vi "Aux DMA FIFO test.vi"() -> ()   [LabVIEW 2019]
uses:
  <vilib>/rvi/Emulation/niFpgaGetClockAttributes.vi
  <vilib>/rvi/Emulation/niFpgaSctlEmulationGetInTimedLoop.vi
  <vilib>/rvi/Emulation/niFpgaEmulationReportErrorSimple.vi
  <vilib>/rvi/eio/common/nirviEmuTemplateMethod_errors.vi
  <vilib>/rvi/Emulation/niFpgaCriticalErrorInLSC.vi
  <vilib>/rvi/interface/RandomDataEmulation/niFpgaRandomDataHandleErrors.vi
  <vilib>/eio/EIONode/EIONode.xnode
  <vilib>/rvi/DataTransferAndStorage/Container/XNode/niFpgaContainer.xnode
  <vilib>/rvi/interface/RandomDataEmulation/nirviRandomDataFpgaReadWriteTemplate.vi
panel:
  in  "xt end aux":u32
  in  "stop":bool
  out "elapsed":u32
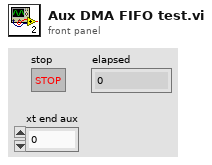
[diagram p1: front panel]
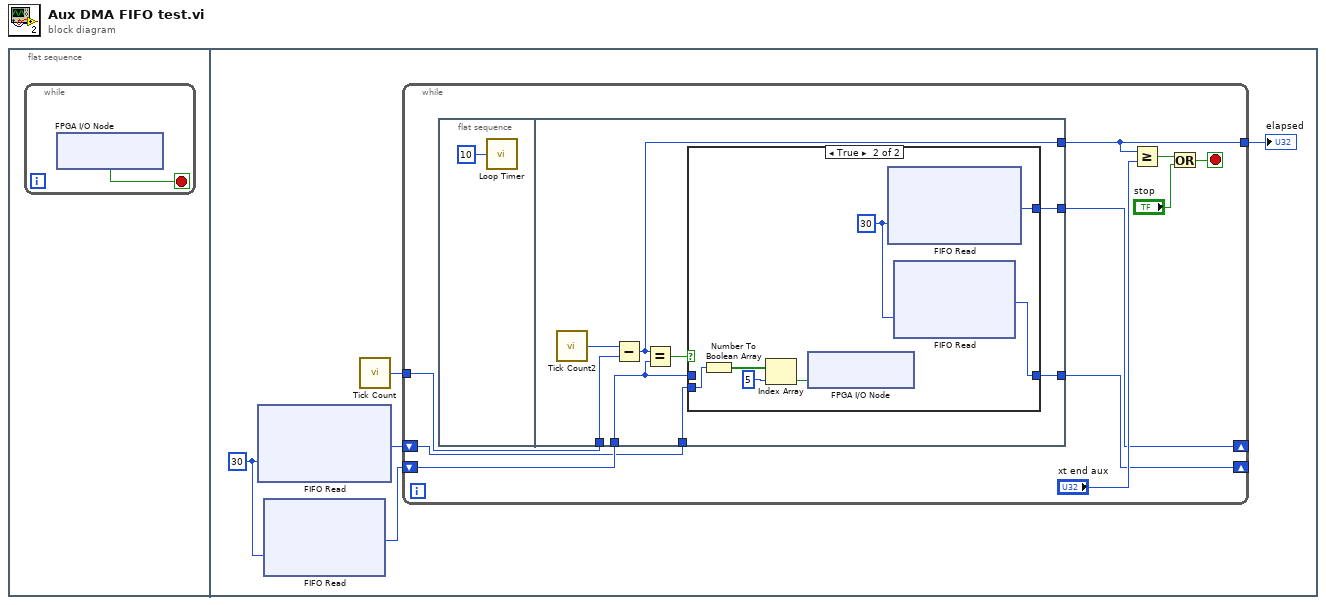
[diagram p0: block diagram]
diagram:
  n1 = flat-sequence {
    frame #0 {
      n2 = while {
        stop <- w1 stop-if-true
        n3 = xnode "FPGA I/O Node"() -> ("RMC/DIO80"=w1:bool)  [unwired: 1 in, 1 out]
      }
    }
    frame #1 {
      w6 = 30 ("Timeout")
      n4 = xnode ("FIFO Read")("Timeout"=w6) -> ("Element"=w4:i16)  [unwired: 1 in, 2 out]
      n5 = xnode ("FIFO Read")("Timeout"=w6) -> ("Element"=w5:i16)  [unwired: 1 in, 2 out]
      n6 = call "Tick Count"() -> ("Tick Count(uSec)"=w3:u32)
      n7 = while {
        shift-right: [w11] -> _
        shift-left: w5 -> [w13]
        shift-right: [w10] -> _
        shift-left: w4 -> [w12]
        tunnel: w3 -> [w14]
        tunnel: [w7] -> w2
        stop <- w8 stop-if-true
        n8 = flat-sequence {
          tunnel: [w23] -> w7
          tunnel: w14 -> [w22]
          tunnel: w13 -> [w18]
          tunnel: w12 -> [w21]
          tunnel: [w20] -> w11
          tunnel: [w19] -> w10
          frame #0 {
            n9 = call "Loop Timer"("Count(Ticks)"=u32 10 ("Count(mSec)")) -> ()  [unwired: 1 out]
          }
          frame #1 {
            n10 = call "Tick Count2"() -> ("Tick Count(uSec)"=w24:u32)
            n11 = Subtract(x=w24, y=w22) -> (x-y=w23:u32)
            n12 = Equal?(x=w23, y=w18) -> (x = y?=w25:bool)
            n13 = case shown="True" w25 {
              tunnel: [w26 w34] -> w19
              tunnel: [w27 w33] -> w20
              tunnel: w21 -> [w26 w31]
              tunnel: w18 -> [w27 _]
              frame False {
              }
              frame True {
                w30 = i16 30
                n14 = Number To Boolean Array(number=w31) -> (Boolean array=w29:bool[])
                n15 = Index Array(array=w29, index=5) -> (element=w28:bool)
                n16 = xnode "FPGA I/O Node"("RMC/DIO83"=w28) -> ()  [unwired: 1 in, 1 out]
                n17 = xnode ("FIFO Read")("Timeout"=w30) -> ("Element"=w34:i16)  [unwired: 1 in, 2 out]
                n18 = xnode ("FIFO Read")("Timeout"=w30) -> ("Element"=w33:i16)  [unwired: 1 in, 2 out]
              }
            }
          }
        }
        n19 = Greater Or Equal?(x=w7, y="xt end aux") -> (x >= y?=w9:bool)
        n20 = Or(x=w9, y="stop") -> (x .or. y?=w8:bool)
      }
      "elapsed" <- w2
    }
  }
